vi "DriveWaitForPiece.vi"(2 "Parameter String":string, 3 "Reinit":bool) -> (0 "Error Out":errorcluster, 1 "Increment":bool)   [LabVIEW 2020]
doc: "This VI pauses the drive sequencer until the driver presses the \"advance system check\" button on the joystick, the joystick will rumble while waiting for the button.\n\nParameters:\nNone"
uses:
  SafeParser_Integer.vi
  GlobalDriverStationCommands.vi
  GlobalGripper.vi
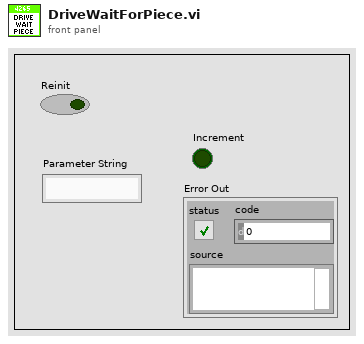
[diagram p1: front panel]
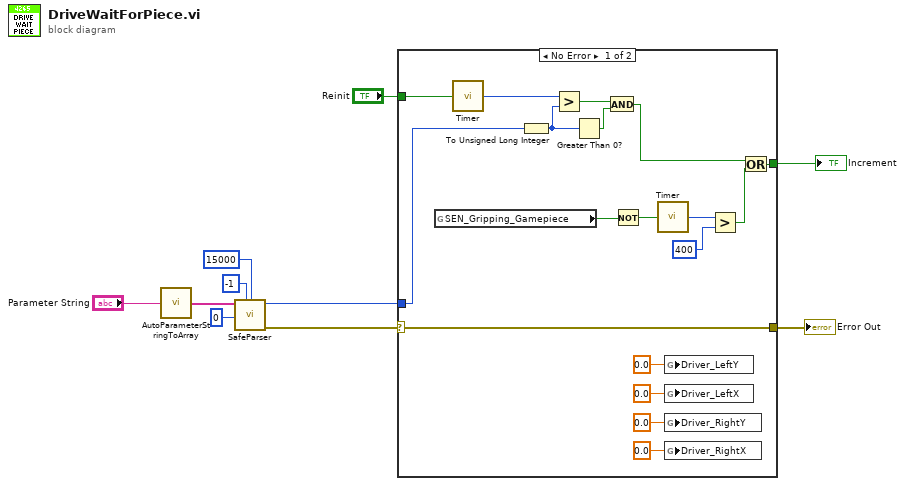
[diagram p0: block diagram]
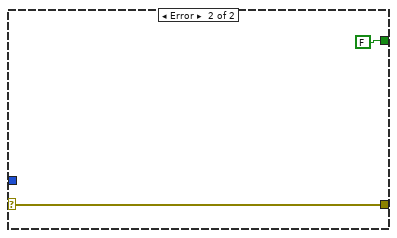
[diagram p2: hidden frame]
diagram:
  n1 = call "AutoParameterStringToArray.vi"("Parameter String"="Parameter String") -> ("Parsed Parameters"=w3:string[])
  n2 = call-poly "SafeParser.vi"("Maximum"=15000, "Minimum"=-1, "Array Index"=0 ("Parameter Index"), "String Array"=w3) -> ("Error Out"=w7:errorcluster, "Typecast  Value"=w8:i32)  [unwired: 6 in]
  n3 = case shown="No Error" w7 {
    selector: w7 -> [w28 w30]
    tunnel: [w23 FALSE] -> w2
    tunnel: "Reinit" -> [w15 _]
    tunnel: [w28 w30] -> w1
    tunnel: w8 -> [w22 _]
    frame No Error {
      n4 = global read "GlobalGripper.vi" "SEN_Gripping_Gamepiece"() -> (w11:bool)
      n5 = call "Timer.vi"("Reset Timer"=w15) -> ("Time (ms)"=w14:u32)
      n6 = To Unsigned Long Integer(number=w22) -> (unsigned 32bit integer=w24:u32)
      n7 = Greater?(x=w14, y=w24) -> (0:w27:bool)
      n8 = Greater Than 0?(x=w24) -> (x > 0?=w26:bool)
      n9 = And(x=w27, y=w26) -> (x .and. y?=w25:bool)
      n10 = Not(x=w11) -> (.not. x?=w13:bool)
      n11 = call "Timer.vi"("Reset Timer"=w13) -> ("Time (ms)"=w12:u32)
      n12 = global write "GlobalDriverStationCommands.vi" "Driver_LeftY"(0.0 ("Driver_LeftY")) -> ()
      n13 = global write "GlobalDriverStationCommands.vi" "Driver_LeftX"(0.0 ("Driver_RightX")) -> ()
      n14 = global write "GlobalDriverStationCommands.vi" "Driver_RightY"(0.0 ("Driver_RightX")) -> ()
      n15 = global write "GlobalDriverStationCommands.vi" "Driver_RightX"(0.0 ("Driver_RightX")) -> ()
      n16 = Greater?(x=w12, y=u32 400) -> (0:w20:bool)
      n17 = Or(x=w25, y=w20) -> (x .or. y?=w23:bool)
    }
    frame Error {
    }
  }
  "Increment" <- w2
  "Error Out" <- w1
